vi "Configure Setpoint and Ramp.vi"(0 "VISA resource name":refnum<visa-resource-name>, 5 "Output's Control Loop (1:1)":u16(ring)=1 items=["1"=1, "2"=2, "3"=3, "4"=4], 7 "Setpoint (0.00000)":dbl format="%.5f", 9 "Setpoint Ramping \nEnable (F: Off)":bool, 11 "error in (no error)":errorcluster, 12 "Ramp Rate (0.0)":dbl format="%.1f") -> (4 "VISA resource name out":refnum<visa-resource-name>, 15 "error out":errorcluster)   [LabVIEW 2012, in "Lake Shore 336.lvlib"]
doc: "This VI configures the Setpoint and Setpoint Ramping function. The Setpoint parameter is used to set the desired load temperature for a control loop."
uses:
  Lake Shore 336.lvlib
  Instance           2 35Saved   Configure Setpoint and Ramp .vi
  Instance           1 35Saved   Configure Setpoint and Ramp .vi
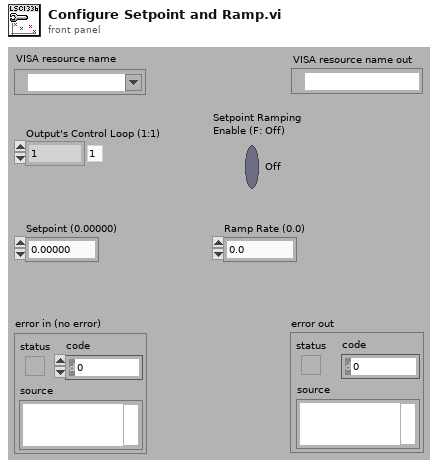
[diagram p1: front panel]
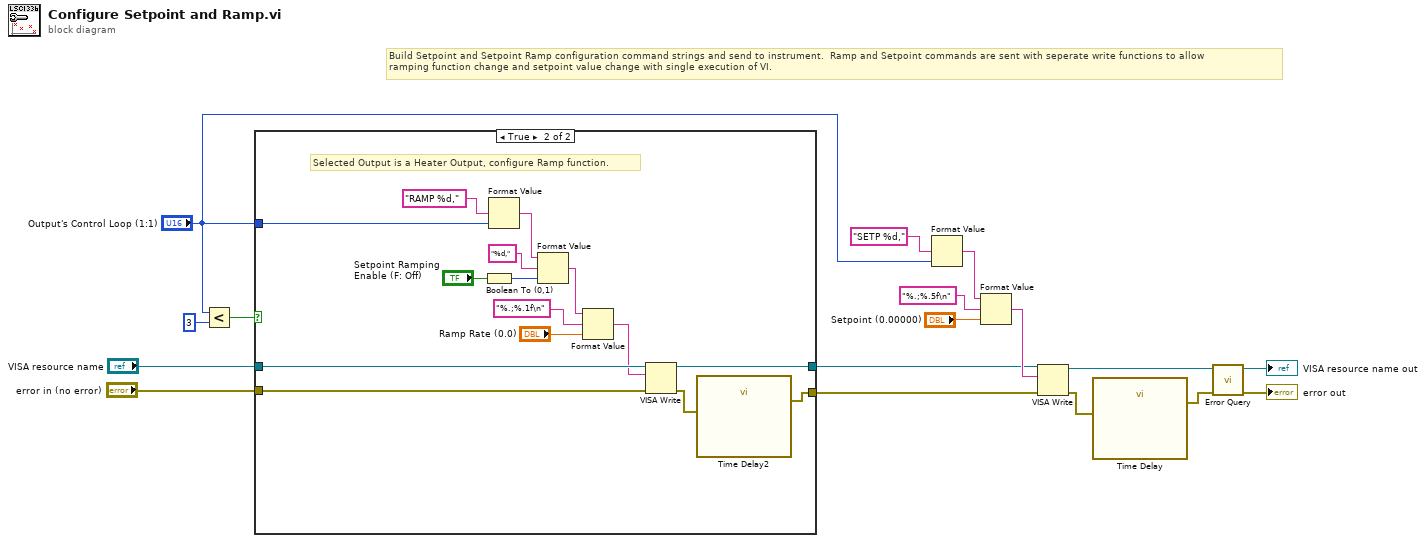
[diagram p0: block diagram]
diagram:
  # "Build Setpoint and Setpoint Ramp configuration command strings and send to instrument.  Ramp and Setpoint commands are sent with seperate write functions to allow\nramping function change and setpoint value change with single execution of VI."
  n1 = Less?(x="Output's Control Loop (1:1)", y=3) -> (x < y?=w5:bool)
  n2 = case shown="True" w5 {
    tunnel: [w19 w27] -> w9
    tunnel: [w18 w26] -> w8
    tunnel: "VISA resource name" -> [w19 w25]
    tunnel: "error in (no error)" -> [w18 w24]
    tunnel: "Output's Control Loop (1:1)" -> [_ w20]
    frame False {
      # "Selected Output is an Unpowered Analog Output, do not configure Ramp function."
    }
    frame True {
      # "Selected Output is a Heater Output, configure Ramp function."
      n3 = Boolean To (0,1)(Boolean="Setpoint Ramping \nEnable (F: Off)") -> (0, 1=w33:i16)
      n4 = Format Value(format string="RAMP %d,", value (0)=w20) -> (output string=w21:string)  [unwired: 1 in]
      n5 = Format Value(string ("")=w21, format string="%d,", value (0)=w33) -> (output string=w31:string)
      n6 = Format Value(string ("")=w31, format string="%.;%.1f\n", value (0)="Ramp Rate (0.0)") -> (output string=w23:string)
      n7 = VISA Write(VISA resource name=w25, write buffer=w23, error in (no error)=w24) -> (VISA resource name out=w27:refnum<visa-resource-name>, error out=w28:errorcluster)  [unwired: 1 out]
      n8 = call "Time Delay2"("error in (no error)"=w28) -> ("error out"=w26:errorcluster)  [unwired: 10 in]
    }
  }
  n9 = Format Value(format string="SETP %d,", value (0)="Output's Control Loop (1:1)") -> (output string=w2:string)  [unwired: 1 in]
  n10 = Format Value(string ("")=w2, format string="%.;%.5f\n", value (0)="Setpoint (0.00000)") -> (output string=w10:string)
  n11 = VISA Write(VISA resource name=w9, write buffer=w10, error in (no error)=w8) -> (VISA resource name out=w17:refnum<visa-resource-name>, error out=w14:errorcluster)  [unwired: 1 out]
  n12 = call "Time Delay"("error in (no error)"=w14) -> ("error out"=w13:errorcluster)  [unwired: 10 in]
  n13 = call "Error Query.vi"("error in (no error)"=w13, "VISA resource name"=w17) -> ("error out"=→"error out":errorcluster, "VISA resource name out"=→"VISA resource name out":refnum<visa-resource-name>)  [unwired: 7 in, 1 out]
